vi "clear_alarm_and_limit_errors.vi"(0 "device_index (in) [0=def]":i32, 2 "axis":T1, 5 "Error In":errorcluster) -> (19 "Error Out":errorcluster)   [LabVIEW 2013, in "examples.lvlib"]
doc: "Produced By:\n\n<B>Kod Integrations, LLC</B>\n4835 Marianne Drive\nMount Airy, MD 21771\nhttp://www.kodintegrations.com\nemail: info@kodintegrations.com\nphone: (240) 687-1288"
uses:
  libraries/examples.lvlib
  classes/Controller/_Controller.lvclass
  common/controls/axis.ctl
  libraries/common.lvlib
panel:
  out "response":string
  out "success?":bool
  in  "clear_buffer? (T)":bool=TRUE
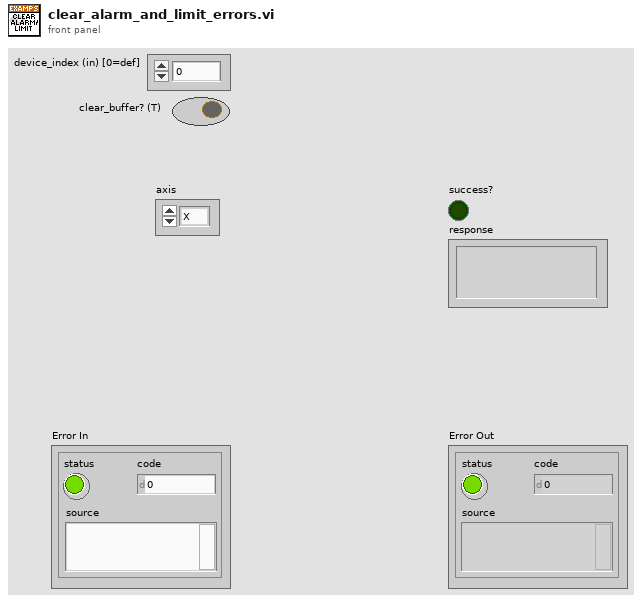
[diagram p1: front panel]
types:
  T1 = typedef "common.lvlib/axis.ctl" = enum16{"X", "Y", "Z", "U"}
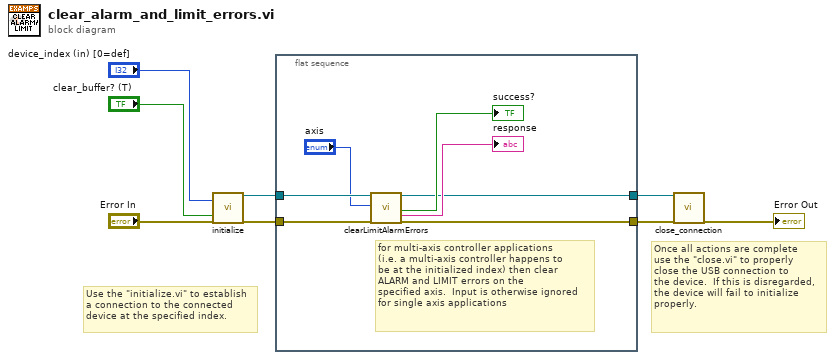
[diagram p0: block diagram]
diagram:
  # "Once all actions are complete\nuse the \"close.vi\" to properly\nclose the USB connection to \nthe device.  If this is disregarded,\nthe device will fail to initialize \nproperly."
  # "Use the \"initialize.vi\" to establish\na connection to the connected\ndevice at the specified index."
  n1 = call "initialize.vi"("device_index (in) [0=def]"="device_index (in) [0=def]", "clear_buffer? (T)"="clear_buffer? (T)", "error in (no error)"="Error In") -> ("reference (out)"=w5:refnum<class "_Controller.lvclass">, "error out"=w4:errorcluster)  [unwired: 15 in]
  n2 = flat-sequence {
    tunnel: w5 -> [w15]
    tunnel: w4 -> [w14]
    tunnel: [w9] -> w3
    tunnel: [w10] -> w2
    frame #0 {
      # "for multi-axis controller applications\n(i.e. a multi-axis controller happens to\nbe at the initialized index) then clear\nALARM and LIMIT errors on the\nspecified axis.  Input is otherwise ignored\nfor single axis applications"
      n3 = call-dynamic "clearLimitAlarmErrors.vi"("Controller in"=w15, "axis"="axis", "error in (no error)"=w14) -> ("Controller out"=w9:refnum<class "_Controller.lvclass">, "success?"=→"success?":bool, "response"=→"response":string, "error out"=w10:errorcluster)  [unwired: 13 in]
    }
  }
  n4 = call "close_connection.vi"("reference (in)"=w3, "error in (no error)"=w2) -> ("error out"=→"Error Out":errorcluster)  [unwired: 16 in, 1 out]
